vi "Messgasverbrauch Anlage.vi"() -> (1 "Ist-Flow":sgl, 3 "Soll-Flow":T1 format="%#_5g")   [LabVIEW 2020, in "allgemeine Sub-VIs.lvlib"]
uses:
  allgemeine Sub-VIs.lvlib
  Visualisierungs Elemente/Zahlen-Eingabefeld.ctl
  Status Analysatoren/Aktion Status Analysatoren.ctl
  Seiten/EL3000/FID/Aktion FGV Messwerte_F.ctl
  Seiten/Anlagengrenzwerte/FGV Anlagengrenzwerte Aktionen.ctl
  Funktionstasten/Funktionstasten-Aktion.ctl
  Funktionstasten/Zustaende.ctl
  cRIO/PC/Kommunikation mit cRIO.lvlib
  Status Analysatoren/Status Analysatoren.lvlib
  Seiten/EL3000/FID/FID.lvlib
  Seiten/Anlagengrenzwerte/Anlagengrenzwerte.lvlib
  Funktionstasten/Funktionstasten.lvlib
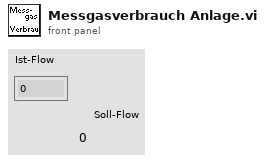
[diagram p1: front panel]
types:
  T1 = typedef "Zahlen-Eingabefeld.ctl" = sgl
  T2 = typedef "Funktionstasten.lvlib/Zustaende.ctl" = enum16{"Standby", "Pause", "Eco", "Messen", "Kalibrieren", "Spülen Filter", "Spülen Leitung", "Umgebungsluft", "0-Gas", "Cal-Gas", "CG zu PNS", "-------------", "Init 1", "Init 2", "Init 3", "Init 4", "Messen vorbereiten", "Messen durchführen", "Exit"}
  T3 = typedef "Funktionstasten.lvlib/Funktionstasten-Aktion.ctl" = enum16{"Initialisieren", "Zustand setzen", "Taste gedrückt", "Fehler speichern", "Lesen", "Manuell", "Remote", "Bitparallel", "Samplepoint", "Zeit Prüfen", "reset Umschalten"}
  T4 = typedef "Anlagengrenzwerte.lvlib/FGV Anlagengrenzwerte Aktionen.ctl" = enum16{"Lesen", "Grenzwerte schreiben"}
  T5 = typedef "ABB-EL3000.lvlib/FID.lvlib/Aktion FGV Messwerte_F.ctl" = enum16{"lesen", "Messwerte", "Messbereich", "Status", "Diagnose Werte"}
  T6 = typedef "Status Analysatoren.lvlib/Aktion Status Analysatoren.ctl" = enum16{"lesen", "initialisieren", "Analysatoren aktiv", "FTIR Fehler", "FID Fehler", "PMA Fehler", "Felder einfärben"}
  T7 = typedef "Verwaltung - cRIO.lvlib/Analog Eingaenge.ctl" = cluster{"AI0: Durchfluss FT-IR":sgl, "AI1: Druck Ausgang":sgl, "AI2: Umgebungsdruck":sgl, "AI3: Druck FT-IR":sgl, "AI4: Druck CalGas":sgl, "AI5: Reserve":sgl, "AI6: Reserve":sgl, "AI7: Reserve":sgl, "Rohwert Durchfluss FT-IR":sgl, "Rohwert Druck Ausgang":sgl, "Rohwert Umgebungsdruck":sgl, "Rohwert Druck FT-IR":sgl, "Rohwert Druck CalGas":sgl, "Rohwert AI5":sgl, "Rohwert AI6":sgl, "Rohwert AI7":sgl, "Rohwert Diffdruck mbar FTIR":sgl}
  T8 = typedef "Anlagengrenzwerte.lvlib/Anlagen-Grenzwerte Anzeige.ctl" = cluster{"Eingangsdruck FT-IR:":T9, "Durchfluss FT-IR:":T9, "Durchfluss CalGas:":T9, "Druck Ausgang:":T9, "Druck Kalter Block:":T9, "Heizleitungen intern:":T9, "Heizleitung zu FT-IR:":T9, "Heizung Filterblock:":T9, "Heizung Pumpe:":T9, "Heizleitung Extern SP1:":T9, "Heizleitung Extern SP2:":T9, "FT-IR Heizung Messzelle:":T9, "Schaltschranktemperatur:":T9, "Gaskühler:":T9}
  T9 = typedef "Anlagengrenzwerte.lvlib/Anlagen-Parameter Anzeige.ctl" = cluster{"Sollwert":sgl, "Warn-Min":sgl, "Warn-Max":sgl, "Abschalt-Min":sgl, "Abschalt-Max":sgl, "Regler":u16}
  T10 = typedef "Status Analysatoren.lvlib/Status.ctl" = cluster{"FT-IR aktiv":bool, "FT-IR Fehler":bool, "FID aktiv":bool, "FID Fehler":bool, "PMA aktiv":bool, "PMA Fehler":bool}
  T11 = cluster{"Temperatur Detektor":sgl, "STG Detektor":sgl, "Temperatur MGE":sgl, "STG MGE":sgl, "Druck Brennluft":sgl, "STG Brennluft":sgl, "Druck Brenngas":sgl, "STG Brenngas":sgl, "Druck MGE":sgl, "STG Druck MGE":sgl, "Druck MGA":sgl, "STG Druck MGA":sgl, "Flow":sgl, "Temperatur Flamme":sgl, "Temperatur NMHC":sgl, "STG NMHC":sgl}
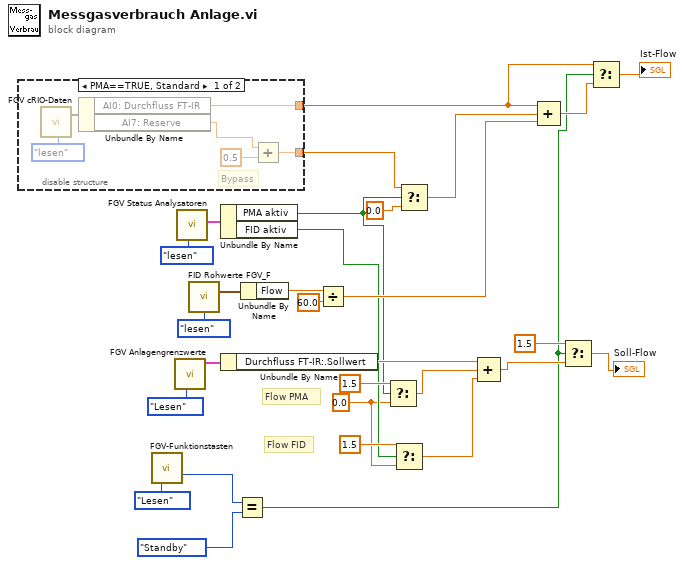
[diagram p0: block diagram]
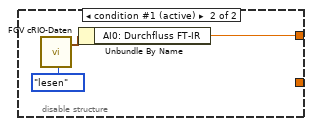
[diagram p2: hidden frame]
diagram:
  w12 = sgl 0.0 ("f")
  # "Flow FID"
  # "Flow PMA"
  n1 = disable-structure shown="PMA==TRUE, Standard" {
    disable-tunnel: [w32 _] -> w11
    disable-tunnel: [w31 w37] -> w1
    frame condition #0 {
      # "Bypass"
      n2 = call "FGV cRIO-Daten.vi"("Aktion"=enum16{"lesen", "schreiben"}."lesen") -> ("Analog Input"=w35:T7)  [unwired: 9 in, 9 out]
      n3 = Unbundle By Name(w35) -> ("AI0: Durchfluss FT-IR"=w31:sgl, "AI7: Reserve"=w33:sgl)
      n4 = Add(x=w33, y=sgl 0.5) -> (x+y=w32:sgl)
    }
    frame condition #1 (active) {
      n5 = call "FGV cRIO-Daten.vi"("Aktion"=enum16{"lesen", "schreiben"}."lesen") -> ("Analog Input"=w38:T7)  [unwired: 9 in, 9 out]
      n6 = Unbundle By Name(w38) -> ("AI0: Durchfluss FT-IR"=w37:sgl)
    }
  }
  n7 = call "FGV-Funktionstasten.vi"("Aktion"=Funktionstasten-Aktion."Lesen") -> ("ausgewählte Funktion"=w9:T2)  [unwired: 7 in, 7 out]
  n8 = call "FGV Anlagengrenzwerte.vi"("Aktion"=FGV_Anlagengrenzwerte_Aktionen."Lesen") -> ("Anlagen-Grenzwerte Anzeige"=w20:T8)  [unwired: 10 in]
  n9 = call "FGV Status Analysatoren.vi"("Aktionen"=Aktion_Status_Analysatoren."lesen") -> ("Status Analysatoren"=w25:T10)  [unwired: 10 in]
  n10 = call "FID Rohwerte FGV_F.vi"("Aktion"=Aktion_FGV_Messwerte_F."lesen") -> ("Diagnose Werte"=w28:T11)  [unwired: 11 in, 3 out]
  n11 = Unbundle By Name(w25) -> ("PMA aktiv"=w16:bool, "FID aktiv"=w13:bool)
  n12 = Unbundle By Name(w20) -> ("Durchfluss FT-IR:.Sollwert"=w19:sgl)
  n13 = Equal?(x=w9, y=Zustaende."Standby") -> (x = y?=w2:bool)
  n14 = Unbundle By Name(w28) -> ("Flow"=w27:sgl)
  n15 = Divide(x=w27, y=sgl 60.0) -> (x/y=w23:sgl)
  n16 = Select(t=sgl 1.5 ("y"), s=w16, f=w12) -> (s? t:f=w18:sgl)
  n17 = Select(t=sgl 1.5 ("y"), s=w13, f=w12) -> (s? t:f=w14:sgl)
  n18 = Select(t=w11, s=w16, f=sgl 0.0) -> (s? t:f=w22:sgl)
  n19 = Compound Arithmetic op=ADD(w19, w18, w14) -> (w5:sgl)
  n20 = Compound Arithmetic op=ADD(w1, w22, w23) -> (w3:sgl)
  n21 = Select(t=sgl 1.5 ("y"), s=w2, f=w5) -> (s? t:f=→"Soll-Flow":sgl)
  n22 = Select(t=w1, s=w2, f=w3) -> (s? t:f=→"Ist-Flow":sgl)
